vi "Load Subpanels.vi"(4 "error in (no error)":errorcluster, 7 "Subpanels to Launch":T1[](array[typedef])) -> (0 "error out":errorcluster)   [LabVIEW 2020, in "Startup Processes.lvlib"]
uses:
  Startup Processes.lvlib
  Config Data/typedefs/Process Launch Data.ctl
  Config Data/typedefs/Process Type.ctl
  toolbox/Timing/Timing.lvlib
  Config Data/Config Data.lvclass
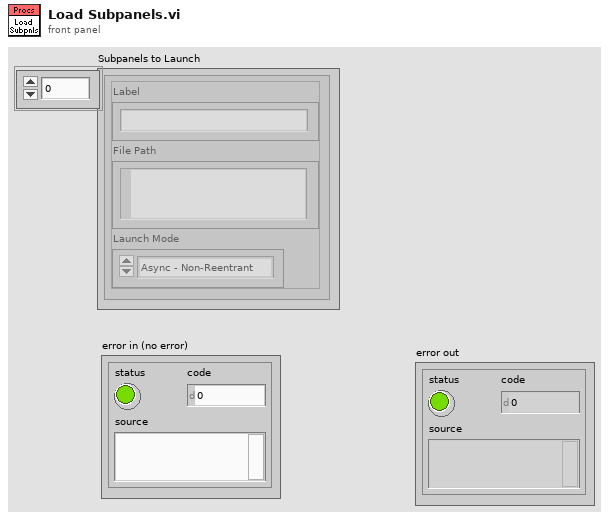
[diagram p1: front panel]
types:
  T1 = typedef "Config Data.lvlib/Config Data.lvclass/Process Launch Data.ctl" = cluster{"Label":string, "File Path":path, "Launch Mode":T2}
  T2 = typedef "Config Data.lvlib/Config Data.lvclass/Process Type.ctl" = enum16{"Async - Non-Reentrant", "Async - Reentrant", "Run Method - Non-Reentrant", "Run Method - Reentrant"}
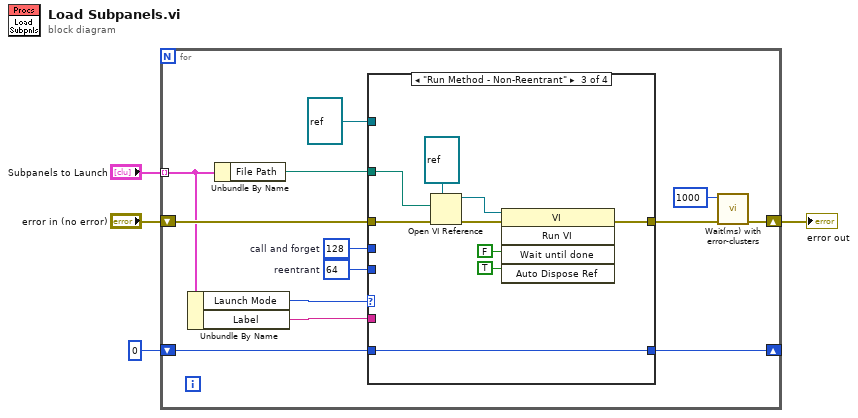
[diagram p0: block diagram]
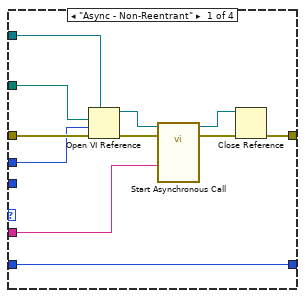
[diagram p2: hidden frame]
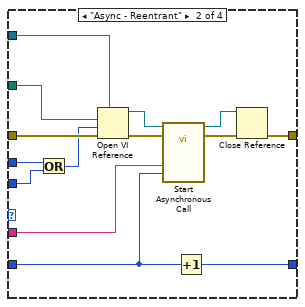
[diagram p3: hidden frame]
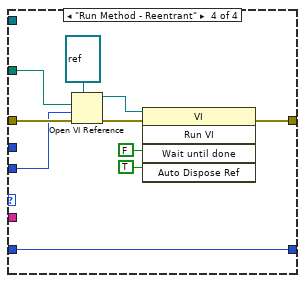
[diagram p4: hidden frame]
diagram:
  n1 = for {
    shift-right: [w11] -> w1
    shift-left: "error in (no error)" -> [w17]
    tunnel: "Subpanels to Launch" -> [w16] mode=indexing
    shift-right: [w5] -> _
    shift-left: 0 -> [w6]
    w7 = 64  # reentrant
    w15 = 128  # call and forget
    n2 = Unbundle By Name(w16) -> ("Launch Mode"=w14:T2, "Label"=w9:string)
    n3 = Unbundle By Name(w16) -> ("File Path"=w13:path)
    n4 = case shown="\"Run Method - Non-Reentrant\"" w14 {
      tunnel: w17 -> [w28 w42 w51 w61]
      tunnel: w13 -> [w27 w41 w50 w60]
      tunnel: w15 -> [w24 w35 _ _]
      tunnel: [w21 w36 w44 w54] -> w12
      tunnel: w9 -> [w18 w29 _ _]
      tunnel: refnum<vi> refnum ("type specifier VI Refnum (for type only)") -> [w20 w33 _ _]
      tunnel: w7 -> [_ w32 _ w53]
      tunnel: w6 -> [w19 w31 w43 w52]
      tunnel: [w19 w30 w43 w52] -> w5
      frame "Async - Non-Reentrant" {
        n5 = Open VI Reference(type specifier VI Refnum (for type only)=w20, vi path=w27, options=w24, error in (no error)=w28) -> (vi reference=w26:refnum<vi>, error out=w25:errorcluster)  [unwired: 2 in]
        n6 = call-by-ref "Start Asynchronous Call"(reference=w26, error in=w25, "My Name"=w18) -> (reference out=w22:refnum<vi>, error out=w23:errorcluster)  [unwired: 11 in]
        n7 = Close Reference(reference=w22, error in (no error)=w23) -> (error out=w21:errorcluster)
      }
      frame "Async - Reentrant" {
        n8 = Or(x=w35, y=w32) -> (x .or. y?=w34:i32)
        n9 = Open VI Reference(type specifier VI Refnum (for type only)=w33, vi path=w41, options=w34, error in (no error)=w42) -> (vi reference=w40:refnum<vi>, error out=w39:errorcluster)  [unwired: 2 in]
        n10 = call-by-ref "Start Asynchronous Call"(reference=w40, error in=w39, "Launch Order"=w31, "My Name"=w29) -> (reference out=w37:refnum<vi>, error out=w38:errorcluster)  [unwired: 10 in]
        n11 = Increment(x=w31) -> (x+1=w30:i32)
        n12 = Close Reference(reference=w37, error in (no error)=w38) -> (error out=w36:errorcluster)
      }
      frame "Run Method - Non-Reentrant" {
        n13 = Open VI Reference(type specifier VI Refnum (for type only)=refnum<vi> refnum, vi path=w50, error in (no error)=w51) -> (vi reference=w48:refnum<vi>, error out=w47:errorcluster)  [unwired: 3 in]
        n14 = invoke class="VI" method="Run VI"(reference=w48, error in=w47, "Wait until done"=FALSE ("Wait Until Done"), "Auto Dispose Ref"=TRUE ("Wait Until Done")) -> (error out=w44:errorcluster)  [unwired: 1 in, 4 out]
      }
      frame "Run Method - Reentrant" {
        n15 = Open VI Reference(type specifier VI Refnum (for type only)=refnum<vi> refnum, vi path=w60, options=w53, error in (no error)=w61) -> (vi reference=w58:refnum<vi>, error out=w57:errorcluster)  [unwired: 2 in]
        n16 = invoke class="VI" method="Run VI"(reference=w58, error in=w57, "Wait until done"=FALSE ("Wait Until Done"), "Auto Dispose Ref"=TRUE ("Wait Until Done")) -> (error out=w54:errorcluster)  [unwired: 1 in, 4 out]
      }
    }
    n17 = call "Wait(ms) with error-clusters.vi"("Error In"=w12, "wait (msec)"=u32 1000 ("milliseconds to wait")) -> ("Error Out"=w11:errorcluster)  [unwired: 5 in]
  }
  "error out" <- w1
